vi "m1m3_getNextSample_HardpointData.vi"(8 "error in (no error)":errorcluster, 11 "HardpointData_Ctl":T1) -> (0 "error out":errorcluster, 2 "function return":i32, 3 "HardpointData_Ctl out":T1)   [LabVIEW 2016, in "SALLV_m1m3.lvlib"]
doc: "int m1m3_shm_getNextSample_HardpointDataLV(m1m3_HardpointDataLV *HardpointData_Ctl );"
uses:
  SALLV_m1m3.lvlib
  DataTypes/HardpointData.ctl
  SALLV_m1m3.so
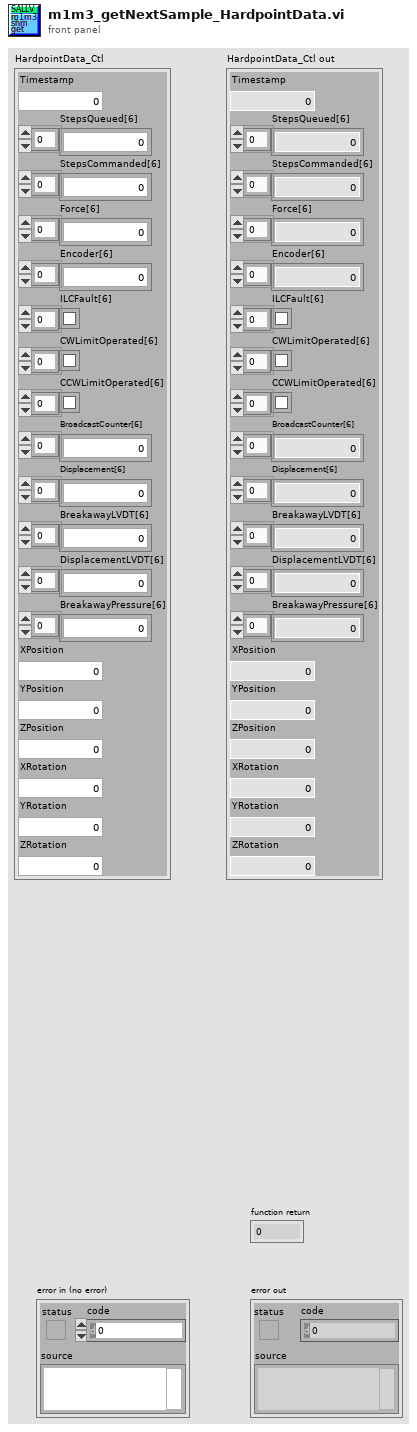
[diagram p1: front panel]
types:
  T1 = typedef "SALLV_m1m3.lvlib/HardpointData.ctl" = cluster{"Timestamp":dbl, "StepsQueued[6]":i32[], "StepsCommanded[6]":i16[], "Force[6]":sgl[], "Encoder[6]":i32[], "ILCFault[6]":bool[], "CWLimitOperated[6]":bool[], "CCWLimitOperated[6]":bool[], "BroadcastCounter[6]":u8[], "Displacement[6]":dbl[], "BreakawayLVDT[6]":sgl[], "DisplacementLVDT[6]":sgl[], "BreakawayPressure[6]":sgl[], "XPosition":dbl, "YPosition":dbl, "ZPosition":dbl, "XRotation":dbl, "YRotation":dbl, "ZRotation":dbl}
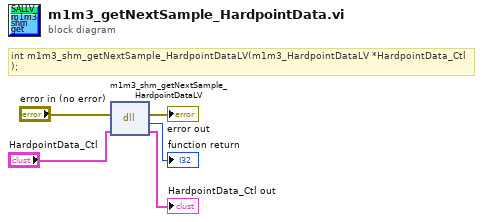
[diagram p0: block diagram]
diagram:
  # "int m1m3_shm_getNextSample_HardpointDataLV(m1m3_HardpointDataLV *HardpointData_Ctl );"
  n1 = dll-call lib="opt/CODE/SALLV_m1m3/SALLV_m1m3.*" fn="m1m3_shm_getNextSample_HardpointDataLV"(error in="error in (no error)", "HardpointData_Ctl"="HardpointData_Ctl") -> (error out=→"error out":errorcluster, →"function return":i32, "HardpointData_Ctl"=→"HardpointData_Ctl out":T1)  [unwired: 2 in, 1 out]
